vi "HW3_stopwatch_2018.vi"() -> ()   [LabVIEW 2018]
panel:
  out "Boolean 2":bool
  out "Boolean":bool
  out "Cluster 7":T1
  out "Cluster 6":T1
  out "Cluster 5":T1
  out "Cluster 4":T1
  out "Cluster 3":T1
  out "Cluster 2":T1
  in  "START/STOP/CLEAR":bool
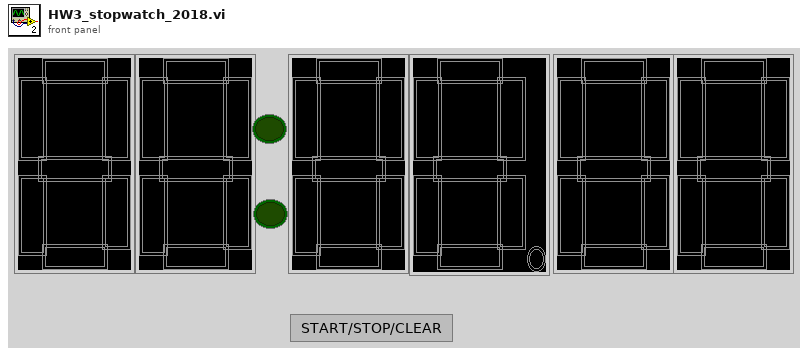
[diagram p1: front panel]
types:
  T1 = cluster{"0":bool, "1":bool, "2":bool, "3":bool, " 4":bool, "5":bool, "6":bool, "p":bool}
  T2 = cluster{"0":bool, "1":bool, "2":bool, "3":bool, " 4":bool, "5":bool, "6":bool, "p":bool}[]
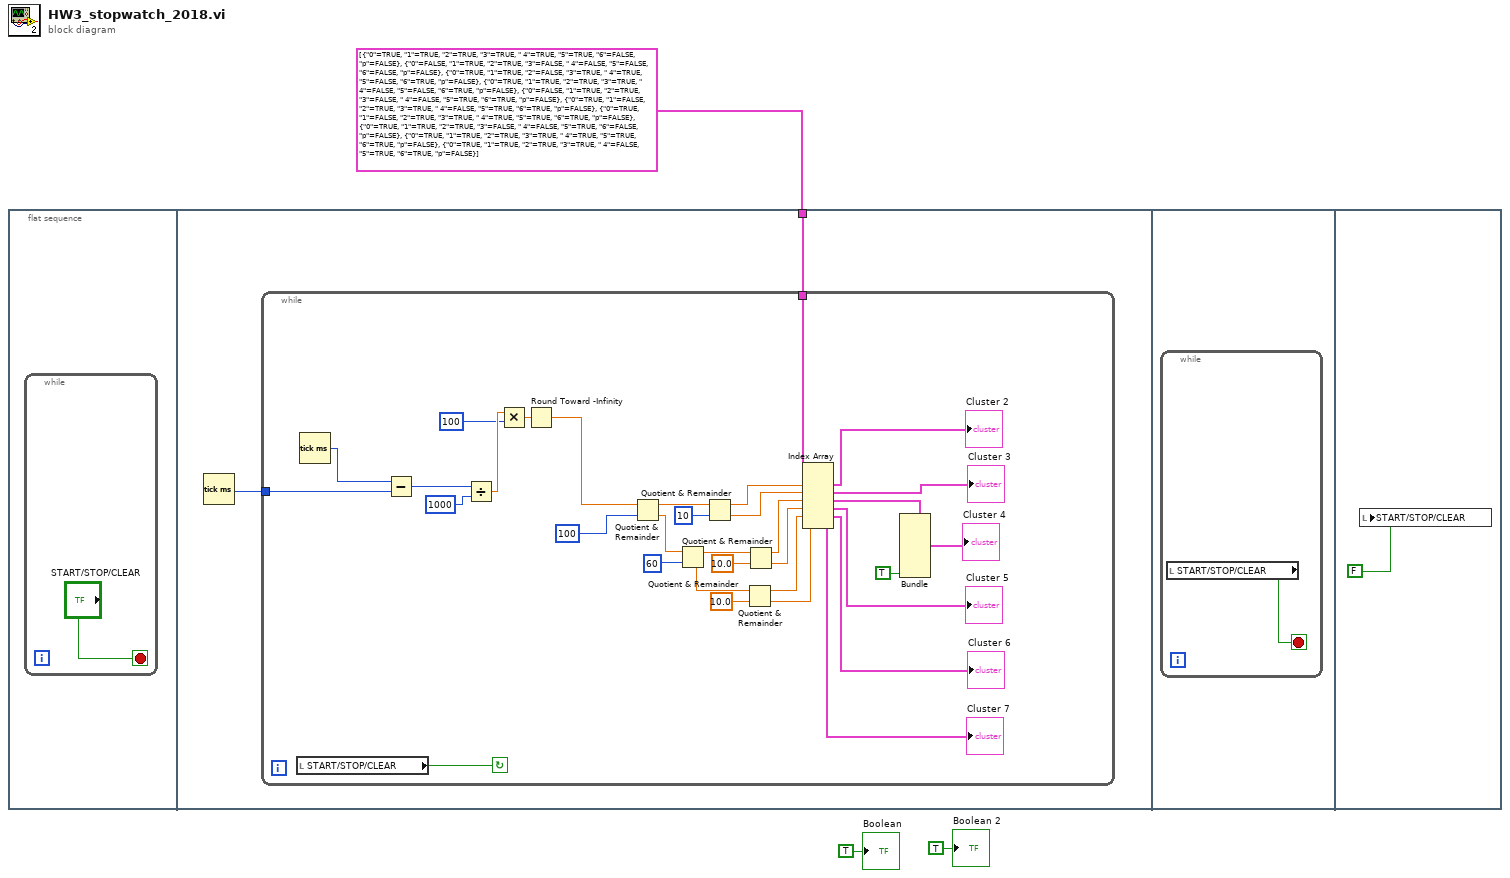
[diagram p0: block diagram]
diagram:
  n1 = flat-sequence {
    tunnel: T2 [{"0"=TRUE, "1"=TRUE, "2"=TRUE, "3"=TRUE, " 4"=TRUE, "5"=TRUE, "6"=FALSE, "p"=FALSE}, {"0"=FALSE, "1"=TRUE, "2"=TRUE, "3"=FALSE, " 4"=FALSE, "5"=FALSE, "6"=FALSE, "p"=FALSE}, {"0"=TRUE, "1"=TRUE, "2"=FALSE, "3"=TRUE, " 4"=TRUE, "5"=FALSE, "6"=TRUE, "p"=FALSE}, {"0"=TRUE, "1"=TRUE, "2"=TRUE, "3"=TRUE, " 4"=FALSE, "5"=FALSE, "6"=TRUE, "p"=FALSE}, {"0"=FALSE, "1"=TRUE, "2"=TRUE, "3"=FALSE, " 4"=FALSE, "5"=TRUE, "6"=TRUE, "p"=FALSE}, {"0"=TRUE, "1"=FALSE, "2"=TRUE, "3"=TRUE, " 4"=FALSE, "5"=TRUE, "6"=TRUE, "p"=FALSE}, {"0"=TRUE, "1"=FALSE, "2"=TRUE, "3"=TRUE, " 4"=TRUE, "5"=TRUE, "6"=TRUE, "p"=FALSE}, {"0"=TRUE, "1"=TRUE, "2"=TRUE, "3"=FALSE, " 4"=FALSE, "5"=TRUE, "6"=FALSE, "p"=FALSE}, {"0"=TRUE, "1"=TRUE, "2"=TRUE, "3"=TRUE, " 4"=TRUE, "5"=TRUE, "6"=TRUE, "p"=FALSE}, {"0"=TRUE, "1"=TRUE, "2"=TRUE, "3"=TRUE, " 4"=FALSE, "5"=TRUE, "6"=TRUE, "p"=FALSE}] -> [w5]
    frame #0 {
      n2 = while {
        stop <- "START/STOP/CLEAR" stop-if-true
      }
    }
    frame #1 {
      n3 = Tick Count (ms)() -> (millisecond timer value=w6:u32)
      n4 = while {
        tunnel: w6 -> [w38]
        tunnel: w5 -> [w20]
        stop <- w35 continue-if-true
        n5 = local read "START/STOP/CLEAR"() -> (w35:bool)
        n6 = Tick Count (ms)() -> (millisecond timer value=w39:u32)
        n7 = Subtract(x=w39, y=w38) -> (x-y=w37:u32)
        n8 = Divide(x=w37, y=1000) -> (x/y=w34:dbl)
        n9 = Multiply(x=w34, y=100) -> (x*y=w32:dbl)
        n10 = Round Toward -Infinity(1:w32) -> (0:w19:dbl)
        n11 = Quotient & Remainder(x=w19, y=100) -> (x-y*floor(x/y)=w26:dbl, floor(x/y)=w16:dbl)
        n12 = Quotient & Remainder(x=w16, y=60) -> (x-y*floor(x/y)=w13:dbl, floor(x/y)=w9:dbl)
        n13 = Quotient & Remainder(x=w26, y=10) -> (x-y*floor(x/y)=w27:dbl, floor(x/y)=w28:dbl)
        n14 = Quotient & Remainder(x=w9, y=10.0) -> (x-y*floor(x/y)=w8:dbl, floor(x/y)=w7:dbl)
        n15 = Quotient & Remainder(x=w13, y=10.0) -> (x-y*floor(x/y)=w12:dbl, floor(x/y)=w11:dbl)
        n16 = Index Array(array=w20, index #1=w27, index #2=w28, index #3=w12, index #4=w11, index #5=w8, index #6=w7) -> (element #1=→"Cluster 2":T1, element #2=→"Cluster 3":T1, element #3=w29:T1, element #4=→"Cluster 5":T1, element #5=→"Cluster 6":T1, element #6=→"Cluster 7":T1)
        n17 = Bundle(cluster=w29, "p"=TRUE) -> (→"Cluster 4":T1)  [unwired: 7 in]
      }
    }
    frame #2 {
      n18 = while {
        stop <- w40 stop-if-true
        n19 = local read "START/STOP/CLEAR"() -> (w40:bool)
      }
    }
    frame #3 {
      n20 = local write "START/STOP/CLEAR"(FALSE ("OK Button")) -> ()
    }
  }
  "Boolean" <- TRUE ("Boolean")
  "Boolean 2" <- TRUE ("Boolean 2")
